vi "Generate Extended Register Read Long Vectors.vi"(0 "Slave Address":T2=12 format="%02x", 1 "Alias":string, 5 "Register Address":T1 format="%02x", 7 "Byte Count":i32=1, 11 "error in (no error)":errorcluster) -> (4 "Vector Statements":string[](array[string]), 15 "error out":errorcluster)   [LabVIEW 2018, in "MIPI RFFE API.lvlib"]
uses:
  MIPI RFFE API.lvlib
  Slave Address.ctl
  Register Address.ctl
  RegReadExtLong/RFFE RegReadExtLong Command.lvclass
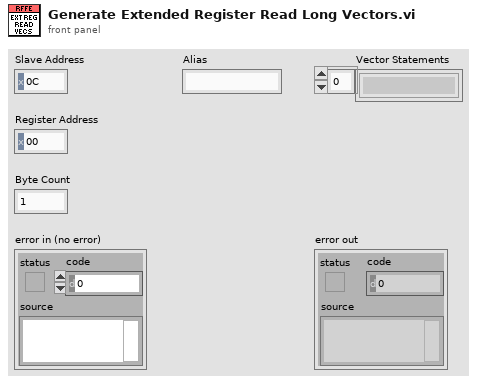
[diagram p1: front panel]
types:
  T1 = typedef "MIPI RFFE API.lvlib/Register Address.ctl" = u16
  T2 = typedef "MIPI RFFE API.lvlib/Slave Address.ctl" = u8
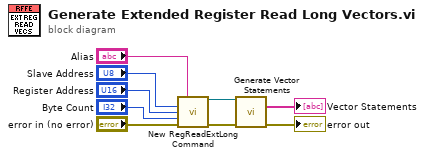
[diagram p0: block diagram]
diagram:
  n1 = call "New RegReadExtLong Command.vi"("Alias"="Alias", "Slave Address"="Slave Address", "Register Address"="Register Address", "Byte Count"="Byte Count", "error in (no error)"="error in (no error)") -> ("RFFE RegReadExtLong Command out"=w5:refnum<class "RFFE RegReadExtLong Command.lvclass">, "error out"=w4:errorcluster)  [unwired: 9 in]
  n2 = call-dynamic "Generate Vector Statements.vi"("RFFE Command in"=w5, "error in (no error)"=w4) -> ("Vector Statements"=→"Vector Statements":string[], "error out"=→"error out":errorcluster)  [unwired: 11 in, 1 out]
